vi "SwrvLinAlg Wheel Core v2.vi"(9 "XY Input":dbl[](array[numeric]), 11 "Wheel":T2(ring)) -> (1 "Debug Outputs":T1, 2 "Drive Output":dbl, 3 "In Range?":bool)   [LabVIEW 2017]
uses:
  SwrvLinAlg Wheel Core Debug Outputs.ctl
  <vilib>/Rock Robotics/WPI/ThirdParty/Phoenix-LabVIEW/Motor Controller/Controls/CTRE_Phoenix_MotorControl_ControlMode.ctl
  Convert Angle to Encoder v2.vi
  Public/Documents/Cross The Road Electronics/Phoenix-LabVIEW/Motor Controller/Get/CTRE_Phoenix_MotorController_GetPulseWidthAll.vi
  <vilib>/Rock Robotics/Network Tables/NT Read Number.vi
  Robot Global Data.vi
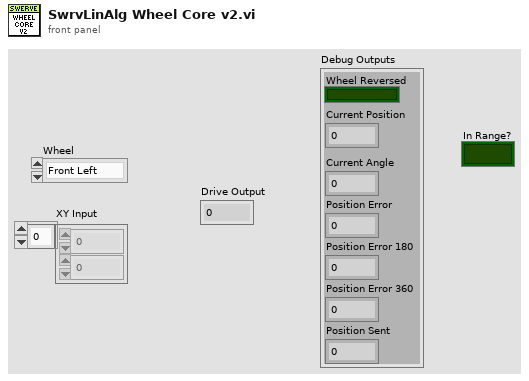
[diagram p1: front panel]
types:
  T1 = typedef "SwrvLinAlg Wheel Core Debug Outputs.ctl" = cluster{"Wheel Reversed":bool, "Current Angle":dbl, "Position Error":dbl, "Position Error 180":dbl, "Position Error 360":dbl, "Position Sent":dbl, "Current Position":dbl}
  T2 = enum16{"Front Left", "Front Right", "Back Left", "Back Right"}
  T3 = typedef "WPI_MotorControlDeviceRef.ctl" = cluster{"DeviceStatus":errorcluster, "Type":T4, "PWM":cluster{"PWM Channel":T5, "DeadBand":T6}, "CAN":cluster{"Device Number":u8, "SetOutput VI Ref":variant, "GetOutput VI Ref":variant, "Enable VI Ref":variant, "Disable VI Ref":variant, "Data":variant}, "Invert":bool, "DIO PWM":cluster{"PWM \"Enable\" Channel":T5, "DIOChannel":T7, "PWM Rate":dbl}}
  T4 = typedef "WPI_MotorControlType.ctl" = enum16{"PWM", "CAN", "DIO PWM"}
  T5 = typedef "FPGA_DIOPWMChannel.ctl" = enum8{"PWM 0", "PWM 1", "PWM 2", "PWM 3", "PWM 4", "PWM 5", "PWM 6", "PWM 7", "PWM 8", "PWM 9", "PWM MXP 0", "PWM MXP 1", "PWM MXP 2", "PWM MXP 3", "PWM MXP 4", "PWM MXP 5", "PWM MXP 6", "PWM MXP 7", "PWM MXP 8", "PWM MXP 9", "Invalid"}
  T6 = typedef "WPI_PWMDeadband.ctl" = cluster{"Name":string, "maxPositivePwm":i32, "minPositivePwm":i32, "centerPwm":i32, "maxNegativePwm":i32, "minNegativePwm":i32, "angularRange":u16}
  T7 = typedef "FPGA_DIOChannel.ctl" = enum8{"DIO 0", "DIO 1", "DIO 2", "DIO 3", "DIO 4", "DIO 5", "DIO 6", "DIO 7", "DIO 8", "DIO 9", "DIO MXP 0", "DIO MXP 1", "DIO MXP 2", "DIO MXP 3", "DIO MXP 4", "DIO MXP 5", "DIO MXP 6", "DIO MXP 7", "DIO MXP 8", "DIO MXP 9", "DIO MXP 10", "DIO MXP 11", "DIO MXP 12", "DIO MXP 13", "DIO MXP 14", "DIO MXP 15", "SPI Port CS1", "SPI Port CS2", "SPI Port CS3", "SPI Port MISO", "SPI Port MOSI", "Invalid"}
  T8 = typedef "CTRE_Phoenix_MotorControl_ControlMode.ctl" = u16
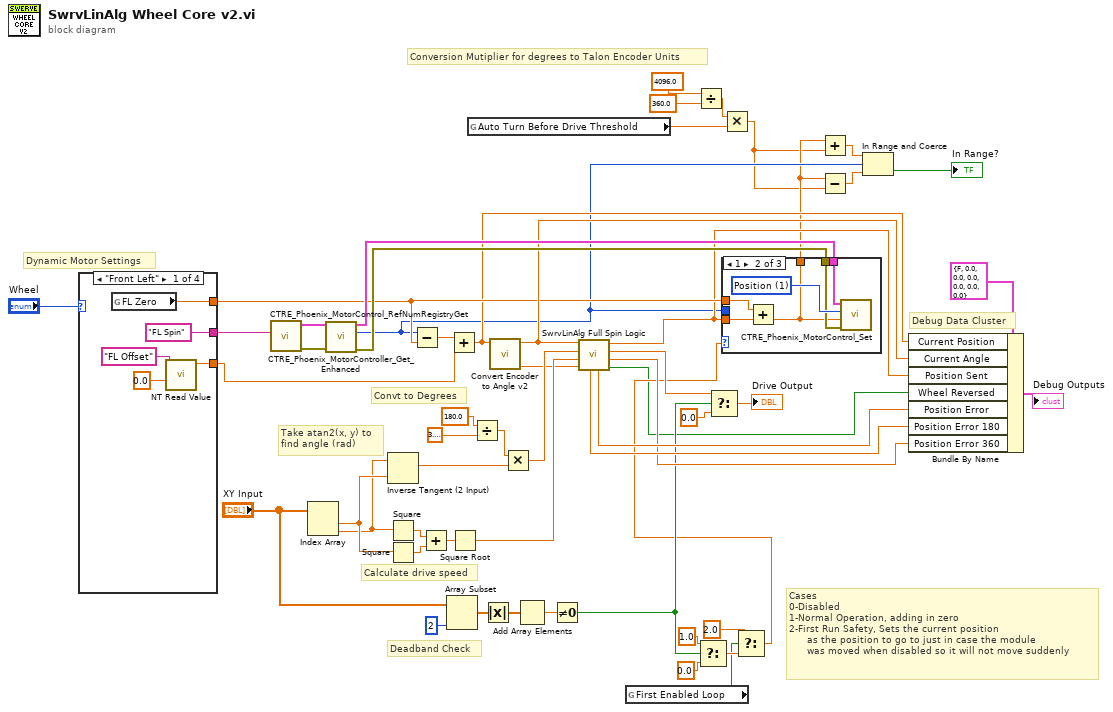
[diagram p0: block diagram]
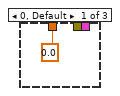
[diagram p2: hidden frame]
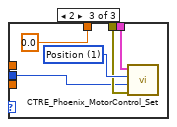
[diagram p3: hidden frame]
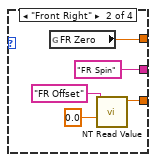
[diagram p4: hidden frame]
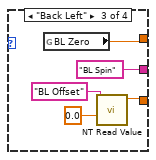
[diagram p5: hidden frame]
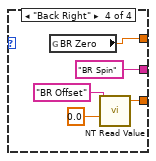
[diagram p6: hidden frame]
diagram:
  # "Cases\n0-Disabled\n1-Normal Operation, adding in zero\n2-First Run Safety, Sets the current position\n      as the position to go to just in case the module\n      was moved when disabled so it will not move suddenly"
  # "Debug Data Cluster"
  # "Conversion Mutiplier for degrees to Talon Encoder Units"
  # "Convt to Degrees"
  # "Take atan2(x, y) to find angle (rad)"
  # "Calculate drive speed"
  # "Deadband Check"
  # "Dynamic Motor Settings"
  n1 = case shown="\"Front Left\"" "Wheel" {
    tunnel: ["FL Spin" ("refnum name") "FR Spin" ("refnum name") "BL Spin" ("refnum name") "BR Spin" ("refnum name")] -> w35
    tunnel: [w57 w62 w67 w72] -> w37
    tunnel: [w56 w61 w66 w71] -> w22
    frame "Front Left" {
      n2 = global read "Robot Global Data.vi" "FL Zero"() -> (w56:dbl)
      n3 = call-poly <vilib>:"NT Read Value.vi"("Default Value"=0.0, "Name"="FL Offset") -> ("Numeric"=w57:dbl)  [unwired: 8 in, 1 out]
    }
    frame "Front Right" {
      n4 = global read "Robot Global Data.vi" "FR Zero"() -> (w61:dbl)
      n5 = call-poly <vilib>:"NT Read Value.vi"("Default Value"=0.0, "Name"="FR Offset") -> ("Numeric"=w62:dbl)  [unwired: 8 in, 1 out]
    }
    frame "Back Left" {
      n6 = global read "Robot Global Data.vi" "BL Zero"() -> (w66:dbl)
      n7 = call-poly <vilib>:"NT Read Value.vi"("Default Value"=0.0, "Name"="BL Offset") -> ("Numeric"=w67:dbl)  [unwired: 8 in, 1 out]
    }
    frame "Back Right" {
      n8 = global read "Robot Global Data.vi" "BR Zero"() -> (w71:dbl)
      n9 = call-poly <vilib>:"NT Read Value.vi"("Default Value"=0.0, "Name"="BR Offset") -> ("Numeric"=w72:dbl)  [unwired: 8 in, 1 out]
    }
  }
  n10 = call "CTRE_Phoenix_MotorControl_RefNumRegistryGet.vi"("refnum name"=w35) -> ("error out"=w53:errorcluster, "PhoenixMotorControlDevRef"=w54:T3)  [unwired: 9 in]
  n11 = Index Array(array="XY Input") -> (element #1=w44:dbl, element #2=w43:dbl)  [unwired: 2 in]
  n12 = call-poly "CTRE_Phoenix_MotorController_Get_Enhanced.vi"("PhoenixMotorControlDevRef"=w54, "error in"=w53) -> ("PhoenixMotorControlDevRef"=w39:T3, "Pulse Width Position"=w10:i32, "error out"=w38:errorcluster)  [unwired: 8 in, 3 out]
  n13 = Inverse Tangent (2 Input)(1:w44, 2:w43) -> (0:w23:dbl)
  n14 = Square(x=w43) -> (x^2=w45:dbl)
  n15 = Square(x=w44) -> (x^2=w48:dbl)
  n16 = Subtract(x=w10, y=w22) -> (x-y=w36:dbl)
  n17 = Add(x=w45, y=w48) -> (x+y=w47:dbl)
  n18 = Array Subset(array="XY Input", length=2) -> (w51:dbl[])  [unwired: 1 in]
  n19 = Add(x=w36, y=w37) -> (x+y=w12:dbl)
  n20 = Square Root(x=w47) -> (sqrt(x)=w40:dbl)
  n21 = global read "Robot Global Data.vi" "Auto Turn Before Drive Threshold"() -> (w4:dbl)
  n22 = Divide(x=180.0 ("y"), y=3.141592653589793) -> (x/y=w46:dbl)
  n23 = Absolute Value(x=w51) -> (abs(x)=w50:dbl[])
  n24 = call "Convert Encoder to Angle v2.vi"("Encoder Units"=w12) -> ("Floor"=w28:dbl, "Angle"=w29:dbl)  [unwired: 9 in]
  n25 = Multiply(x=w46, y=w23) -> (x*y=w42:dbl)
  n26 = Add Array Elements(numeric array=w50) -> (sum=w49:dbl)
  n27 = Not Equal To 0?(x=w49) -> (x != 0?=w16:bool)
  n28 = call "SwrvLinAlg Full Spin Logic.vi"("E>A Floor"=w28, "Drive Wheel"=w40, "Target Angle"=w42, "Current Encoder Angle"=w29) -> ("Wheel Reversed"=w14:bool, "Position Error 360"=w26:dbl, "Adjusted Drive"=w31:dbl, "Spin Wheel Command"=w11:dbl, "Position Error"=w33:dbl, "Position Error 180"=w32:dbl)  [unwired: 2 in]
  n29 = global read "Robot Global Data.vi" "First Enabled Loop"() -> (w17:bool)
  n30 = Divide(x=4096.0, y=360.0) -> (x/y=w5:dbl)
  n31 = Select(t=1.0, s=w16, f=0.0) -> (s? t:f=w20:dbl)
  n32 = Select(t=w31, s=w16, f=0.0) -> (s? t:f=→"Drive Output":dbl)
  n33 = Multiply(x=w5, y=w4) -> (x*y=w1:dbl)
  n34 = Select(t=2.0, s=w17, f=w20) -> (s? t:f=w15:dbl)
  n35 = case shown="1" w15 {
    tunnel: w39 -> [_ w81 w86]
    tunnel: w38 -> [_ w80 w85]
    tunnel: w11 -> [_ w79 _]
    tunnel: w22 -> [_ w78 _]
    tunnel: w10 -> [_ _ w84]
    tunnel: [0.0 w77 0.0] -> w7
    frame 0, Default {
    }
    frame 1 {
      w82 = T8 1 items=["PercentOutput"=0, "Position"=1, "Velocity"=2, "Current"=3, "Follower"=5, "MotionProfile"=6, "MotionMagic"=7, "MotionMagicArc"=8, "MotionProfileArc"=10, "Disabled"=15] ("Control Mode")
      n36 = Add(x=w78, y=w79) -> (x+y=w77:dbl)
      n37 = call <vilib>:"CTRE_Phoenix_MotorControl_Set.vi"("error in (no error)"=w80, "Output"=w77, "Control Mode"=w82, "PhoenixMotorControlDevRef"=w81) -> ()  [unwired: 6 in, 2 out]
    }
    frame 2 {
      w87 = T8 1 items=["PercentOutput"=0, "Position"=1, "Velocity"=2, "Current"=3, "Follower"=5, "MotionProfile"=6, "MotionMagic"=7, "MotionMagicArc"=8, "MotionProfileArc"=10, "Disabled"=15] ("Control Mode")
      n38 = call <vilib>:"CTRE_Phoenix_MotorControl_Set.vi"("error in (no error)"=w85, "Output"=w84, "Control Mode"=w87, "PhoenixMotorControlDevRef"=w86) -> ()  [unwired: 6 in, 2 out]
    }
  }
  n39 = Add(x=w7, y=w1) -> (x+y=w9:dbl)
  n40 = Subtract(x=w7, y=w1) -> (x-y=w8:dbl)
  n41 = In Range and Coerce(upper limit=w9, x=w10, lower limit=w8) -> (In Range?=→"In Range?":bool)  [unwired: 1 out]
  n42 = Bundle By Name(cluster=T1 {"Wheel Reversed"=FALSE, "Current Angle"=0.0, "Position Error"=0.0, "Position Error 180"=0.0, "Position Error 360"=0.0, "Position Sent"=0.0, "Current Position"=0.0} ("Wheel Core Debug Outputs"), "Current Position"=w12, "Current Angle"=w29, "Position Sent"=w11, "Wheel Reversed"=w14, "Position Error"=w33, "Position Error 180"=w32, "Position Error 360"=w26) -> (→"Debug Outputs":T1)
